vi "MotorControl.vi"() -> ()   [LabVIEW 2013]
doc: "<B>Motor Control.vi</B> demonstrates simplistic control of a motor using PWM."
uses:
  <vilib>/Rock Robotics/SystemInterfaces/Typedef/FPGA_TypedefDigitalModule.ctl
  <vilib>/Rock Robotics/SystemInterfaces/DIO/FPGA_DIOPWMChannel.ctl
  <vilib>/Rock Robotics/WPI/Joystick/WPI_JoystickDeviceEnum.ctl
  <vilib>/Rock Robotics/WPI/MotorControl/WPI_MotorControlOpen Talon.vi
panel:
  out "Victor LED":bool
  in  "PWM Channel":T1
  in  "DIO Module":T2
  in  "stop":bool
  # "Wiring Diagram for Digital Sidecar connected to an NI 9403"
  # "Set these inputs before running."
  # "This can be set while running."
  # "Digital Sidecar"
  # "Power\nTerminals"
  # "Motor\nTerminals"
  # "PWM cable"
  # "This shows wiring for a Victor speed controller.  The wiring is similar for a Luminary Micro Jaguar speed controller.  For a Jaguar, you must also select the appropriate instance of the Motor Open VI on the diagram."
  # "V-"
  # "M-"
  # "V+"
  # "M+"
  # "B"
  # "Innovation First"
  # "VICTOR 884"
  # "B"
  # "C"
  # "PWR"
  # "SIG"
  # "(-)"
  # "+V"
  # "10"
  # "9"
  # "8"
  # "7"
  # "6"
  # "5"
  # "4"
  # "3"
  # "2"
  # "1"
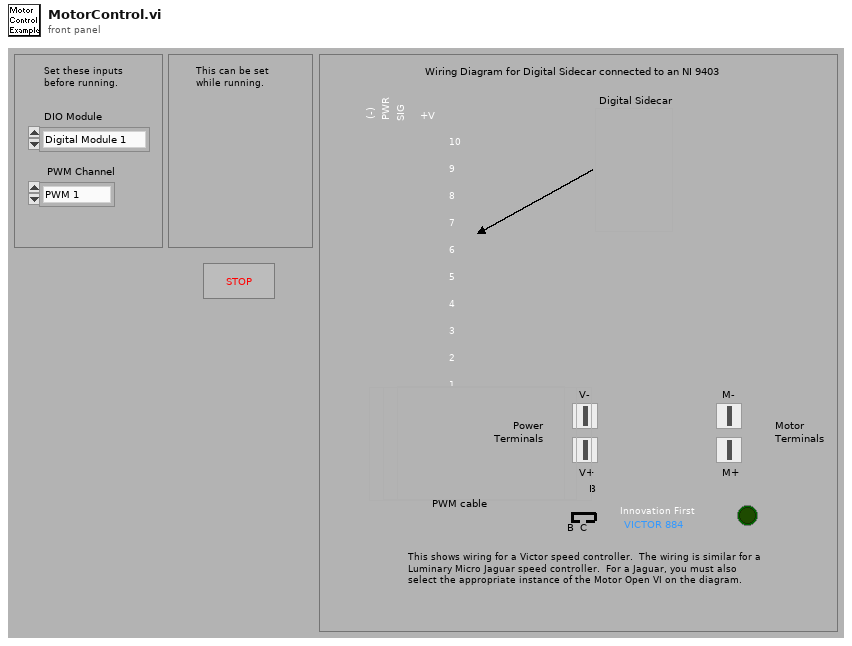
[diagram p1: front panel]
types:
  T1 = typedef "FPGA_DIOPWMChannel.ctl" = enum8{"PWM 1", "PWM 2", "PWM 3", "PWM 4", "PWM 5", "PWM 6", "PWM 7", "PWM 8", "PWM 9", "PWM 10", "Invalid"}
  T2 = typedef "FPGA_TypedefDigitalModule.ctl" = enum16{"Digital Module 1", "Digital Module 2"}
  T3 = typedef "WPI_JoystickDeviceEnum.ctl" = enum16{"USB 1", "USB 2", "USB 3", "USB 4", "Kinect 1", "Kinect 2"}
  T4 = typedef "WPI_MotorControlDeviceRef.ctl" = cluster{"DeviceStatus":errorcluster, "Type":enum16{"PWM", "CAN"}, "PWM":cluster{"Digital Module":T2, "PWM Channel":T1, "DeadBand":T5}, "CAN":cluster{"Device Number":u8, "Control Mode":T6, "Semaphore":T7, "Max Vout":dbl}, "Invert":bool, "TransformRef":T8, "InvTransformRef":T8}
  T5 = typedef "WPI_PWMDeadband.ctl" = cluster{"Name":string, "maxPositivePwm":i32, "minPositivePwm":i32, "centerPwm":i32, "maxNegativePwm":i32, "minNegativePwm":i32, "angularRange":u16}
  T6 = typedef "WPI_CANJaguar_ControlMode.ctl" = enum8{"Percent VBus", "Current", "Speed", "Position", "Voltage"}
  T7 = typedef "Semaphore RefNum" = refnum<k1>
  T8 = typedef "WPI_PWMTransform_ConPane.ctl" = refnum<vi>
  T9 = typedef "WPI_JoystickDevRef.ctl" = cluster{"Device":T3}
  T10 = cluster{"axis 1 (x)":dbl, "axis 2 (y)":dbl, "axis 3 (throttle)":dbl, "axis 4":dbl, "axis 5":dbl, "axis 6":dbl}
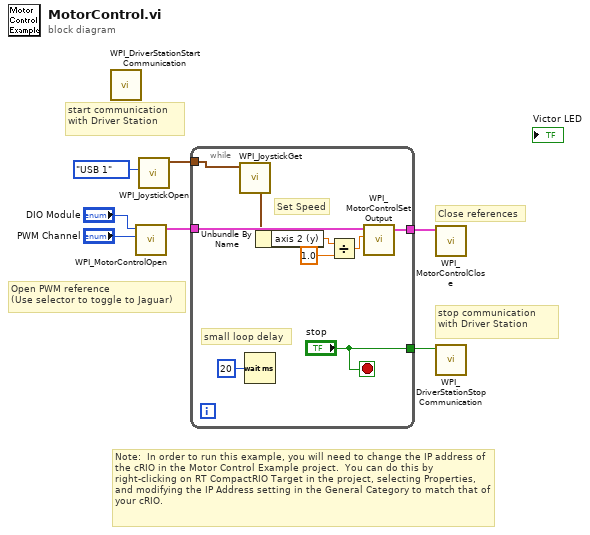
[diagram p0: block diagram]
diagram:
  # "stop communication with Driver Station"
  # "start communication with Driver Station"
  # "Note:  In order to run this example, you will need to change the IP address of the cRIO in the Motor Control Example project.  You can do this by right-clicking on RT CompactRIO Target in the project, selecting Properties, and modifying the IP Address setting in the General Category to match that of your cRIO."
  # "Close references"
  # "Open PWM reference\n(Use selector to toggle to Jaguar)"
  n1 = call <vilib>:"WPI_DriverStationStart Communication.vi"() -> ()  [unwired: 1 in, 11 out]
  n2 = call-poly <vilib>:"WPI_MotorControlOpen.vi"("PWM Channel"="PWM Channel", "Digital Module (Module 1)"="DIO Module") -> ("MotorControlDeviceRef"=w5:T4)  [unwired: 5 in, 4 out]
  n3 = call <vilib>:"WPI_JoystickOpen.vi"("JoystickDevice"=WPI_JoystickDeviceEnum."USB 1") -> ("JoystickDevRef"=w1:T9)  [unwired: 10 in]
  n4 = while {
    tunnel: w5 -> [w16]
    tunnel: [w15] -> w4
    tunnel: ["stop"] -> w3
    tunnel: w1 -> [w12]
    stop <- "stop" stop-if-true
    # "small loop delay"
    # "Set Speed"
    n5 = call <vilib>:"WPI_JoystickGet.vi"("JoystickDevRef"=w12) -> ("Axes"=w11:T10)  [unwired: 4 in, 2 out]
    n6 = Wait (ms)(milliseconds to wait=u32 20) -> ()  [unwired: 1 out]
    n7 = Unbundle By Name(w11) -> ("axis 2 (y)"=w10:dbl)
    n8 = Divide(x=w10, y=1.0) -> (x/y=w8:dbl)
    n9 = call <vilib>:"WPI_MotorControlSetOutput.vi"("Output"=w8, "MotorControlDevRef"=w16) -> ("MotorControlDevRef"=w15:T4)  [unwired: 3 in, 6 out]
  }
  n10 = call <vilib>:"WPI_MotorControlClose.vi"("MotorControlDevRef"=w4) -> ()  [unwired: 1 in, 10 out]
  n11 = call <vilib>:"WPI_DriverStationStop Communication.vi"("StopCommunication"=w3) -> ()  [unwired: 1 in, 10 out]
